vi "CRYCalc Wave & Constant.vi"(0 "Wave in":T1={"Waveform"={"X0"=0.0, "dX"=0.0, "Y"=[]}, "X data"=1, "Y data"=1, "Y axis"=1, "X unit"="s", "Y unit"="V", "Y dB ref"=1.0, "display Y"=TRUE, "display X"=TRUE, "Overload?"=FALSE, "Test Info"="", "Step No."=0, "Name"="", "protected"=FALSE, "Sqc history"=[], "Signal Channel ID"=0, "Plot Settings"={"Color"=0, "Interpolation"=0, "Point Style"=0, "Line Style"=0, "Point Color"=0, "Line Width"=0, "Bar Plot Style"=0, "Fill To"=0}, "AutoProtect"=FALSE} {"Y dB ref" format="%.1f"; "Y axis" items=["Log", "Lin"]; "Y data" items=["dB", "Lin"]; "X data" items=["dB", "Lin"]}, 5 "Value in":T2={"Name"="", "Curve"=[], "X data"=1, "Y data"=1, "Z data"=1, "X axis"=0, "Y axis"=1, "Z axis"=1, "X unit"="Hz", "Y unit"="", "Z unit"="deg.", "X dB ref"=1.0, "Y dB ref"=1.0, "Z dB ref"=1.0, "single val"=FALSE, "protected"=FALSE, "display X"=TRUE, "display Y"=TRUE, "display Z"=TRUE, "Test Info"="", "Step No."=0, "Plot Settings"={"Color"=0, "Interpolation"=0, "Point Style"=0, "Line Style"=0, "Point Color"=0, "Line Width"=0, "Bar Plot Style"=0, "Fill To"=0}, "AutoProtect"=FALSE} {"Z data" items=["dB", "Lin"]; "X data" items=["dB", "Lin"]; "Y data" items=["dB", "Lin"]; "Z dB ref" format="%.1f"; "Z axis" items=["Log", "Lin"]; "X dB ref" format="%.1f"; "X axis" items=["Log", "Lin"]; "Y axis" items=["Log", "Lin"]; "Y dB ref" format="%.1f"; "Curve"."z" format="%.2f"; "Curve"."y" format="%.2f"; "Curve"."x" format="%.2f"}, 7 "Operator":u16(ring) items=["+", "--", "x", "/"], 9 "Work in":u16(slide), 11 "A_axis mode":u16(slide) scale=0.0..2.0, 12 "B_axis mode":u16(slide) scale=0.0..2.0, 13 "Constant":dbl) -> (4 "Wave out":T1={"Waveform"={"X0"=0.0, "dX"=0.0, "Y"=[]}, "X data"=1, "Y data"=1, "Y axis"=1, "X unit"="s", "Y unit"="V", "Y dB ref"=1.0, "display Y"=TRUE, "display X"=TRUE, "Overload?"=FALSE, "Test Info"="", "Step No."=0, "Name"="", "protected"=FALSE, "Sqc history"=[], "Signal Channel ID"=0, "Plot Settings"={"Color"=0, "Interpolation"=0, "Point Style"=0, "Line Style"=0, "Point Color"=0, "Line Width"=0, "Bar Plot Style"=0, "Fill To"=0}, "AutoProtect"=FALSE} {"Y dB ref" format="%.1f"; "Y axis" items=["Log", "Lin"]; "Y data" items=["dB", "Lin"]; "X data" items=["dB", "Lin"]})   [LabVIEW 2013]
uses:
  Typedef Control/CRYData Cluster.ctl
  Typedef Control/CRYWaveform Cluster.ctl
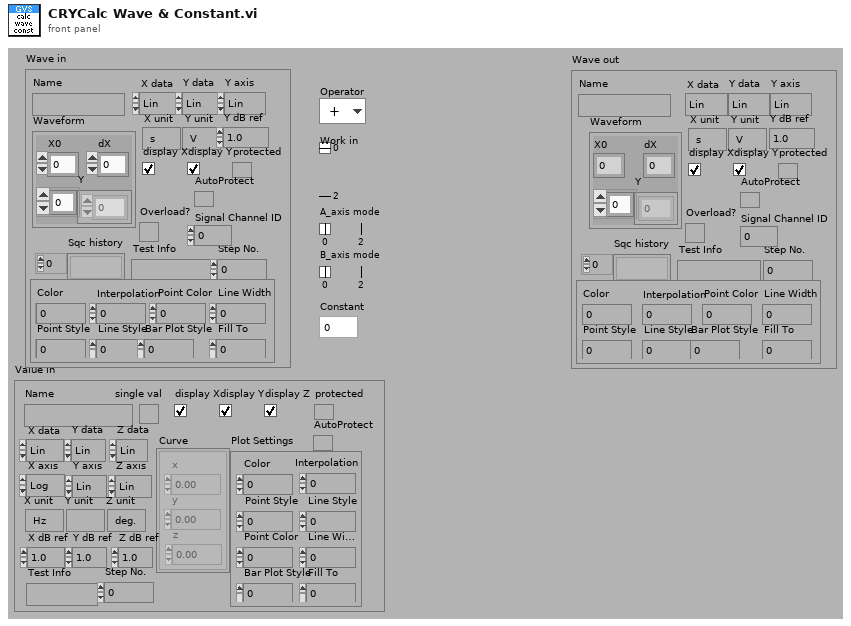
[diagram p1: front panel]
types:
  T1 = typedef "CRYWaveform Cluster.ctl" = cluster{"Waveform":cluster{"X0":dbl, "dX":dbl, "Y":sgl[]}, "X data":u16, "Y data":u16, "Y axis":u16, "X unit":string, "Y unit":string, "Y dB ref":dbl, "display Y":bool, "display X":bool, "Overload?":bool, "Test Info":string, "Step No.":i32, "Name":string, "protected":bool, "Sqc history":string[], "Signal Channel ID":i32, "Plot Settings":cluster{"Color":u32, "Interpolation":u8, "Point Style":u8, "Line Style":u8, "Point Color":u32, "Line Width":u8, "Bar Plot Style":u8, "Fill To":i16}, "AutoProtect":bool}
  T2 = typedef "CRYData Cluster.ctl" = cluster{"Name":string, "Curve":cluster{"x":dbl, "y":dbl, "z":dbl}[], "X data":u16, "Y data":u16, "Z data":u16, "X axis":u16, "Y axis":u16, "Z axis":u16, "X unit":string, "Y unit":string, "Z unit":string, "X dB ref":dbl, "Y dB ref":dbl, "Z dB ref":dbl, "single val":bool, "protected":bool, "display X":bool, "display Y":bool, "display Z":bool, "Test Info":string, "Step No.":i32, "Plot Settings":cluster{"Color":u32, "Interpolation":u8, "Point Style":u8, "Line Style":u8, "Point Color":u32, "Line Width":u8, "Bar Plot Style":u8, "Fill To":i16}, "AutoProtect":bool}
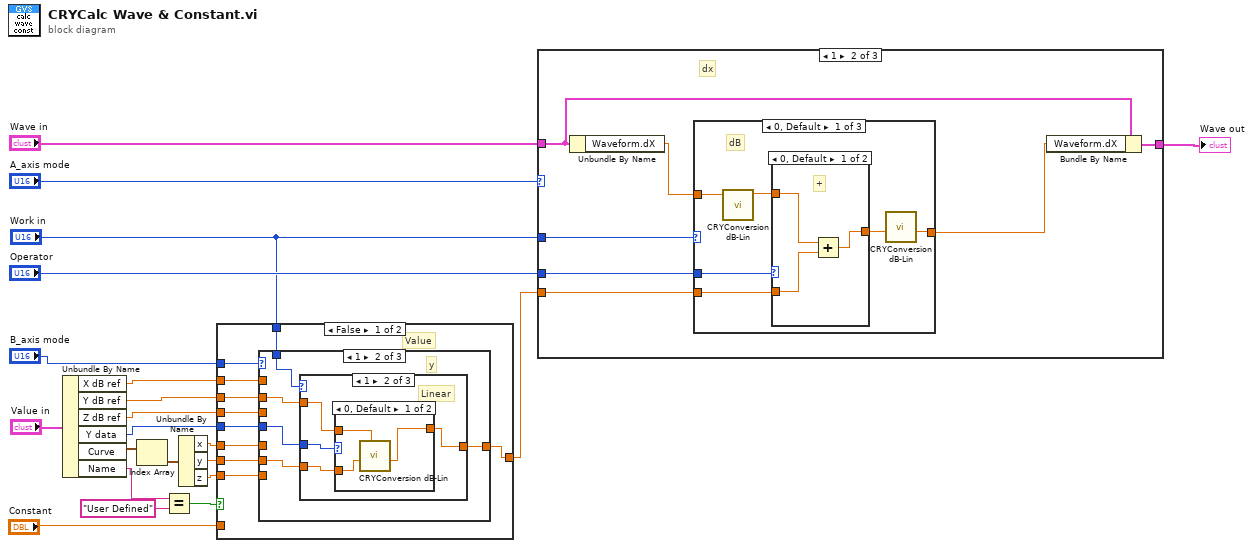
[diagram p0: block diagram]
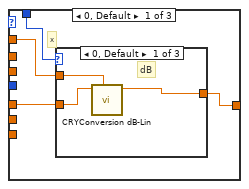
[diagram p2: hidden frame]
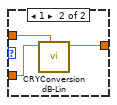
[diagram p6: hidden frame]
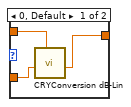
[diagram p9: hidden frame]
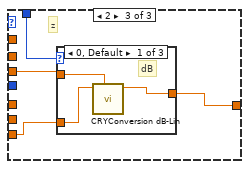
[diagram p10: hidden frame]
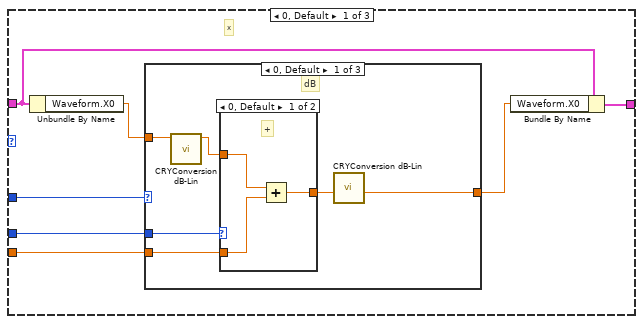
[diagram p14: hidden frame]
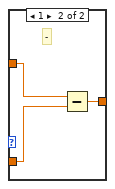
[diagram p15: hidden frame]
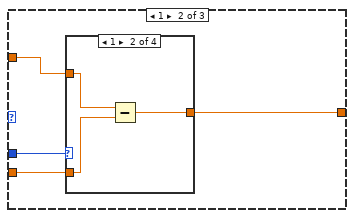
[diagram p16: hidden frame]
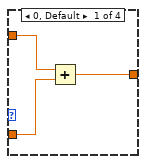
[diagram p17: hidden frame]
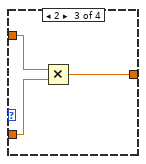
[diagram p18: hidden frame]
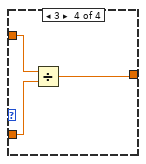
[diagram p19: hidden frame]
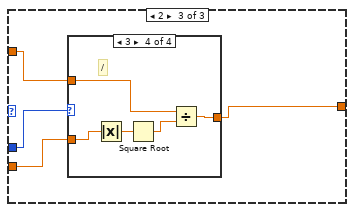
[diagram p20: hidden frame]
diagram:
  n1 = Unbundle By Name("Value in") -> ("X dB ref"=w12:dbl, "Y dB ref"=w13:dbl, "Z dB ref"=w14:dbl, "Y data"=w15:u16, "Curve"=w17:cluster{"x":dbl, "y":dbl, "z":dbl}[], "Name"=w10:string)
  n2 = Index Array(array=w17) -> (element=w16:cluster{"x":dbl, "y":dbl, "z":dbl})  [unwired: 1 in]
  n3 = Equal?(x=w10, y="User Defined") -> (x = y?=w11:bool)
  n4 = Unbundle By Name(w16) -> ("x"=w7:dbl, "y"=w6:dbl, "z"=w5:dbl)
  n5 = case shown="False" w11 {
    tunnel: "Constant" -> [_ w79]
    tunnel: "B_axis mode" -> [w31 _]
    tunnel: w12 -> [w25 _]
    tunnel: w13 -> [w24 _]
    tunnel: w14 -> [w23 _]
    tunnel: w15 -> [w22 _]
    tunnel: w7 -> [w30 _]
    tunnel: w6 -> [w28 _]
    tunnel: w5 -> [w27 _]
    tunnel: [w29 w79] -> w3
    tunnel: "Work in" -> [w26 _]
    frame False {
      # "Value"
      n6 = case shown="1" w31 {
        tunnel: [w32 w42 w70] -> w29
        tunnel: w30 -> [w33 _ _]
        tunnel: w28 -> [_ w44 _]
        tunnel: w27 -> [_ _ w71]
        tunnel: w26 -> [w34 w43 w73]
        tunnel: w25 -> [w35 _ _]
        tunnel: w24 -> [_ w45 _]
        tunnel: w23 -> [_ _ w72]
        tunnel: w22 -> [_ w41 _]
        frame 0, Default {
          # "x"
          n7 = case shown="0, Default" w34 {
            tunnel: w35 -> [w38 _ _]
            tunnel: w33 -> [w37 w39 w40]
            tunnel: [w36 w39 w40] -> w32
            frame 0, Default {
              # "dB"
              n8 = call "CRYConversion dB-Lin.vi"("dB ref."=w38, "Lin In"=w37) -> ("Log Out"=w36:dbl)  [unwired: 4 in, 3 out]
            }
            frame 1 {
              # "Linear"
            }
            frame 2 {
              # "Power"
            }
          }
        }
        frame 1 {
          # "y"
          n9 = case shown="1" w43 {
            tunnel: w45 -> [w46 w55 w65]
            tunnel: w44 -> [w48 w56 w63]
            tunnel: [w47 w54 w62] -> w42
            tunnel: w41 -> [w49 w57 w64]
            frame 0, Default {
              # "dB"
              n10 = case shown="0, Default" w49 {
                tunnel: [w50 w51] -> w47
                tunnel: w48 -> [w50 w52]
                tunnel: w46 -> [_ w53]
                frame 0, Default {
                }
                frame 1 {
                  n11 = call "CRYConversion dB-Lin.vi"("dB ref."=w53, "Lin In"=w52) -> ("Log Out"=w51:dbl)  [unwired: 4 in, 3 out]
                }
              }
            }
            frame 1 {
              # "Linear"
              n12 = case shown="0, Default" w57 {
                tunnel: [w58 w61] -> w54
                tunnel: w56 -> [w59 w61]
                tunnel: w55 -> [w60 _]
                frame 0, Default {
                  n13 = call "CRYConversion dB-Lin.vi"("dB ref."=w60, "Log In"=w59) -> ("Lin Out"=w58:dbl)  [unwired: 4 in, 3 out]
                }
                frame 1 {
                }
              }
            }
            frame 2 {
              # "Power"
              n14 = case shown="1" w64 {
                tunnel: [w67 w69] -> w62
                tunnel: w63 -> [w66 w69]
                tunnel: w65 -> [w68 _]
                frame 0, Default {
                  n15 = call "CRYConversion dB-Lin.vi"("dB ref."=w68, "Log In"=w66) -> ("Lin Out"=w67:dbl)  [unwired: 4 in, 3 out]
                }
                frame 1 {
                }
              }
            }
          }
        }
        frame 2 {
          # "z"
          n16 = case shown="0, Default" w73 {
            tunnel: w72 -> [w76 _ _]
            tunnel: w71 -> [w75 w77 w78]
            tunnel: [w74 w77 w78] -> w70
            frame 0, Default {
              # "dB"
              n17 = call "CRYConversion dB-Lin.vi"("dB ref."=w76, "Lin In"=w75) -> ("Log Out"=w74:dbl)  [unwired: 4 in, 3 out]
            }
            frame 1 {
              # "Linear"
            }
            frame 2 {
              # "Power"
            }
          }
        }
      }
    }
    frame True {
    }
  }
  n18 = case shown="1" "A_axis mode" {
    tunnel: "Wave in" -> [w83 w143 w205]
    tunnel: "Operator" -> [w86 w145 w207]
    tunnel: w3 -> [w85 w144 w206]
    tunnel: "Work in" -> [w81 w146 w208]
    tunnel: [w80 w142 w204] -> w18
    frame 0, Default {
      # "x"
      n19 = Unbundle By Name(w83) -> ("Waveform.X0"=w84:dbl)
      n20 = case shown="0, Default" w81 {
        tunnel: w86 -> [w92 w102 w118]
        tunnel: w85 -> [w91 w100 w116]
        tunnel: w84 -> [w90 w101 w117]
        tunnel: [w87 w99 w115] -> w82
        frame 0, Default {
          # "dB"
          n21 = call "CRYConversion dB-Lin.vi"("Lin In"=w90) -> ("Log Out"=w89:dbl)  [unwired: 5 in, 3 out]
          n22 = case shown="0, Default" w92 {
            tunnel: w91 -> [w94 w96]
            tunnel: w89 -> [w95 w97]
            tunnel: [w93 w98] -> w88
            frame 0, Default {
              # "+"
              n23 = Add(x=w95, y=w94) -> (x+y=w93:dbl)
            }
            frame 1 {
              # "-"
              n24 = Subtract(x=w97, y=w96) -> (x-y=w98:dbl)
            }
          }
          n25 = call "CRYConversion dB-Lin.vi"("Log In"=w88) -> ("Lin Out"=w87:dbl)  [unwired: 5 in, 3 out]
        }
        frame 1 {
          n26 = case shown="1" w102 {
            tunnel: w101 -> [w105 w108 w111 w113]
            tunnel: w100 -> [w104 w107 w110 w112]
            tunnel: [w103 w106 w109 w114] -> w99
            frame 0, Default {
              n27 = Add(x=w105, y=w104) -> (x+y=w103:dbl)
            }
            frame 1 {
              n28 = Subtract(x=w108, y=w107) -> (x-y=w106:dbl)
            }
            frame 2 {
              n29 = Multiply(x=w111, y=w110) -> (x*y=w109:dbl)
            }
            frame 3 {
              n30 = Divide(x=w113, y=w112) -> (x/y=w114:dbl)
            }
          }
        }
        frame 2 {
          n31 = case shown="3" w118 {
            tunnel: w117 -> [w124 w131 w134 w139]
            tunnel: w116 -> [w123 w130 w136 w141]
            tunnel: [w119 w125 w135 w140] -> w115
            frame 0, Default {
              # "+"
              n32 = Square(x=w124) -> (x^2=w122:dbl)
              n33 = Square(x=w123) -> (x^2=w121:dbl)
              n34 = Add(x=w122, y=w121) -> (x+y=w120:dbl)
              n35 = Square Root(x=w120) -> (sqrt(x)=w119:dbl)
            }
            frame 1 {
              # "-"
              n36 = Square(x=w131) -> (x^2=w129:dbl)
              n37 = Square(x=w130) -> (x^2=w128:dbl)
              n38 = Subtract(x=w129, y=w128) -> (x-y=w127:dbl)
              n39 = Absolute Value(x=w127) -> (abs(x)=w126:dbl)
              n40 = Square Root(x=w126) -> (sqrt(x)=w125:dbl)
            }
            frame 2 {
              # "*"
              n41 = Absolute Value(x=w136) -> (abs(x)=w132:dbl)
              n42 = Square Root(x=w132) -> (sqrt(x)=w133:dbl)
              n43 = Multiply(x=w134, y=w133) -> (x*y=w135:dbl)
            }
            frame 3 {
              # "/"
              n44 = Absolute Value(x=w141) -> (abs(x)=w137:dbl)
              n45 = Square Root(x=w137) -> (sqrt(x)=w138:dbl)
              n46 = Divide(x=w139, y=w138) -> (x/y=w140:dbl)
            }
          }
        }
      }
      n47 = Bundle By Name(cluster=w83, "Waveform.X0"=w82) -> (w80:T1)
    }
    frame 1 {
      # "dx"
      n48 = Unbundle By Name(w143) -> ("Waveform.dX"=w148:dbl)
      n49 = case shown="0, Default" w146 {
        tunnel: w145 -> [w152 w162 w177]
        tunnel: w144 -> [w150 w163 w179]
        tunnel: w148 -> [w151 w164 w180]
        tunnel: [w149 w161 w178] -> w147
        frame 0, Default {
          # "dB"
          n50 = call "CRYConversion dB-Lin.vi"("Lin In"=w151) -> ("Log Out"=w153:dbl)  [unwired: 5 in, 3 out]
          n51 = case shown="0, Default" w152 {
            tunnel: w150 -> [w156 w158]
            tunnel: w153 -> [w157 w159]
            tunnel: [w155 w160] -> w154
            frame 0, Default {
              # "+"
              n52 = Add(x=w157, y=w156) -> (x+y=w155:dbl)
            }
            frame 1 {
              # "-"
              n53 = Subtract(x=w159, y=w158) -> (x-y=w160:dbl)
            }
          }
          n54 = call "CRYConversion dB-Lin.vi"("Log In"=w154) -> ("Lin Out"=w149:dbl)  [unwired: 5 in, 3 out]
        }
        frame 1 {
          n55 = case shown="1" w162 {
            tunnel: w164 -> [w167 w170 w173 w175]
            tunnel: w163 -> [w166 w169 w172 w174]
            tunnel: [w165 w168 w171 w176] -> w161
            frame 0, Default {
              n56 = Add(x=w167, y=w166) -> (x+y=w165:dbl)
            }
            frame 1 {
              n57 = Subtract(x=w170, y=w169) -> (x-y=w168:dbl)
            }
            frame 2 {
              n58 = Multiply(x=w173, y=w172) -> (x*y=w171:dbl)
            }
            frame 3 {
              n59 = Divide(x=w175, y=w174) -> (x/y=w176:dbl)
            }
          }
        }
        frame 2 {
          n60 = case shown="0, Default" w177 {
            tunnel: w180 -> [w186 w193 w196 w201]
            tunnel: w179 -> [w185 w192 w198 w203]
            tunnel: [w181 w187 w197 w202] -> w178
            frame 0, Default {
              # "+"
              n61 = Square(x=w186) -> (x^2=w184:dbl)
              n62 = Square(x=w185) -> (x^2=w183:dbl)
              n63 = Add(x=w184, y=w183) -> (x+y=w182:dbl)
              n64 = Square Root(x=w182) -> (sqrt(x)=w181:dbl)
            }
            frame 1 {
              # "-"
              n65 = Square(x=w193) -> (x^2=w191:dbl)
              n66 = Square(x=w192) -> (x^2=w190:dbl)
              n67 = Subtract(x=w191, y=w190) -> (x-y=w189:dbl)
              n68 = Absolute Value(x=w189) -> (abs(x)=w188:dbl)
              n69 = Square Root(x=w188) -> (sqrt(x)=w187:dbl)
            }
            frame 2 {
              # "*"
              n70 = Absolute Value(x=w198) -> (abs(x)=w194:dbl)
              n71 = Square Root(x=w194) -> (sqrt(x)=w195:dbl)
              n72 = Multiply(x=w196, y=w195) -> (x*y=w197:dbl)
            }
            frame 3 {
              # "/"
              n73 = Absolute Value(x=w203) -> (abs(x)=w199:dbl)
              n74 = Square Root(x=w199) -> (sqrt(x)=w200:dbl)
              n75 = Divide(x=w201, y=w200) -> (x/y=w202:dbl)
            }
          }
        }
      }
      n76 = Bundle By Name(cluster=w143, "Waveform.dX"=w147) -> (w142:T1)
    }
    frame 2 {
      # "y"
      n77 = Unbundle By Name(w205) -> ("Waveform.Y"=w210:sgl[])
      n78 = for {
        tunnel: w210 -> [w215] mode=indexing
        tunnel: [w214] -> w209 mode=indexing
        tunnel: w208 -> [w213]
        tunnel: w207 -> [w212]
        tunnel: w206 -> [w211]
        n79 = case shown="0, Default" w213 {
          tunnel: w212 -> [w225 w239 w255]
          tunnel: w211 -> [w224 w237 w254]
          tunnel: w215 -> [w220 w238 w253]
          tunnel: [w217 w236 w252] -> w214
          frame 0, Default {
            # "dB"
            n80 = Absolute Value(x=w220) -> (abs(x)=w221:sgl)
            n81 = call "CRYConversion dB-Lin.vi"("Lin In"=w221) -> ("Log Out"=w222:dbl)  [unwired: 5 in, 3 out]
            n82 = case shown="0, Default" w225 {
              tunnel: w224 -> [w231 w233]
              tunnel: w222 -> [w232 w234]
              tunnel: [w230 w235] -> w223
              frame 0, Default {
                n83 = Add(x=w232, y=w231) -> (x+y=w230:dbl)
              }
              frame 1 {
                n84 = Subtract(x=w234, y=w233) -> (x-y=w235:dbl)
              }
            }
            n85 = call "CRYConversion dB-Lin.vi"("Log In"=w223) -> ("Lin Out"=w216:dbl)  [unwired: 5 in, 3 out]
            n86 = Greater?(x=w220, y=sgl 0.0) -> (0:w218:bool)
            n87 = case shown="False" w218 {
              tunnel: [w228 w229] -> w217
              tunnel: w216 -> [w227 w229]
              frame False {
                n88 = Multiply(x=-1.0, y=w227) -> (x*y=w228:dbl)
              }
              frame True {
              }
            }
          }
          frame 1 {
            # "lin"
            n89 = case shown="0, Default" w239 {
              tunnel: w238 -> [w242 w245 w248 w250]
              tunnel: w237 -> [w241 w244 w247 w249]
              tunnel: [w240 w243 w246 w251] -> w236
              frame 0, Default {
                # "+"
                n90 = Add(x=w242, y=w241) -> (x+y=w240:dbl)
              }
              frame 1 {
                # "-"
                n91 = Subtract(x=w245, y=w244) -> (x-y=w243:dbl)
              }
              frame 2 {
                # "*"
                n92 = Multiply(x=w248, y=w247) -> (x*y=w246:dbl)
              }
              frame 3 {
                # "/"
                n93 = Divide(x=w250, y=w249) -> (x/y=w251:dbl)
              }
            }
          }
          frame 2 {
            # "pow"
            n94 = case shown="3" w255 {
              tunnel: w253 -> [w261 w268 w271 w276]
              tunnel: w254 -> [w260 w267 w273 w278]
              tunnel: [w256 w262 w272 w277] -> w252
              frame 0, Default {
                # "+"
                n95 = Square(x=w261) -> (x^2=w259:sgl)
                n96 = Square(x=w260) -> (x^2=w258:dbl)
                n97 = Add(x=w259, y=w258) -> (x+y=w257:dbl)
                n98 = Square Root(x=w257) -> (sqrt(x)=w256:dbl)
              }
              frame 1 {
                # "-"
                n99 = Square(x=w268) -> (x^2=w266:sgl)
                n100 = Square(x=w267) -> (x^2=w265:dbl)
                n101 = Subtract(x=w266, y=w265) -> (x-y=w264:dbl)
                n102 = Absolute Value(x=w264) -> (abs(x)=w263:dbl)
                n103 = Square Root(x=w263) -> (sqrt(x)=w262:dbl)
              }
              frame 2 {
                # "*"
                n104 = Absolute Value(x=w273) -> (abs(x)=w269:dbl)
                n105 = Square Root(x=w269) -> (sqrt(x)=w270:dbl)
                n106 = Multiply(x=w271, y=w270) -> (x*y=w272:dbl)
              }
              frame 3 {
                # "/"
                n107 = Absolute Value(x=w278) -> (abs(x)=w274:dbl)
                n108 = Square Root(x=w274) -> (sqrt(x)=w275:dbl)
                n109 = Divide(x=w276, y=w275) -> (x/y=w277:dbl)
              }
            }
          }
        }
      }
      n110 = Bundle By Name(cluster=w205, "Waveform.Y"=w209) -> (w204:T1)
    }
  }
  "Wave out" <- w18
